vi "Close.vi"(8 "error in (no error)":errorcluster, 11 "Network Device in":refnum<class "Network Device.lvclass">) -> (0 "error out":errorcluster, 3 "Network Device out":refnum<class "Network Device.lvclass">)   [LabVIEW 2013, in "Network Device.lvclass"]
uses:
  Network Device.lvclass
  VISA/VISA.lvclass/VISA.ctl
  VISA/Read Ref.vi
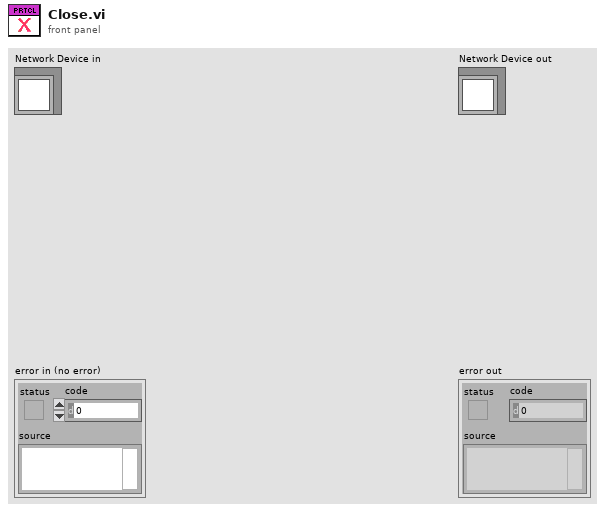
[diagram p1: front panel]
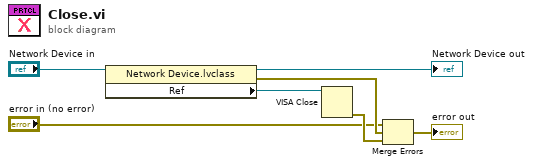
[diagram p0: block diagram]
diagram:
  n1 = property class="Network Device.lvclass"(reference="Network Device in") -> (reference out=→"Network Device out":refnum<class "Network Device.lvclass">, error out=w5:errorcluster, "Ref"=w7:refnum<visa-resource-name>)  [unwired: 1 in]
  n2 = VISA Close(VISA resource name=w7) -> (error out=w6:errorcluster)  [unwired: 1 in]
  n3 = Merge Errors("error in (no error)", w5, w6) -> (→"error out":errorcluster)
